vi "Write Process.Trigger.vi"(8 "error in":errorcluster, 10 "Process.Trigger":refnum<k33>, 11 "Process in":refnum<class "Process.lvclass">) -> (0 "error out":errorcluster, 3 "Process out":refnum<class "Process.lvclass">)   [LabVIEW 2024, in "VS Plugin Inline Async API.lvlib" / "Process.lvclass"]
uses:
  Process.lvclass
  Process.lvclass/Process.ctl
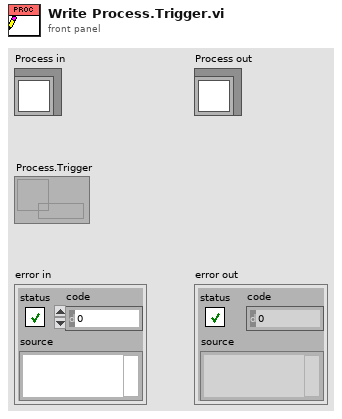
[diagram p1: front panel]
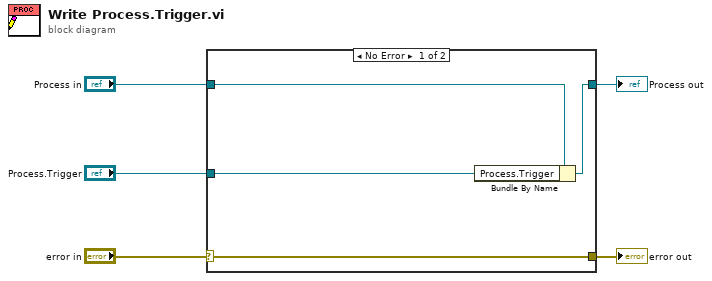
[diagram p0: block diagram]
diagram:
  n1 = case shown="No Error" "error in" {
    selector: "error in" -> [w9 w11]
    tunnel: [w9 w11] -> w4
    tunnel: [w7 w10] -> w2
    tunnel: "Process in" -> [w8 w10]
    tunnel: "Process.Trigger" -> [w6 _]
    frame No Error {
      n2 = Bundle By Name(cluster=w8, "Process.Trigger"=w6) -> (w7:refnum<class "Process.lvclass">)
    }
    frame Error {
    }
  }
  "error out" <- w4
  "Process out" <- w2
